vi "setFPGA.vi"(10 "FPGA":refnum<class "FPGA.lvclass">, 11 "ModbusSubnetETxDataFIFO in":refnum<class "ModbusSubnetETxDataFIFO.lvclass">) -> (3 "ModbusSubnetETxDataFIFO out":refnum<class "ModbusSubnetETxDataFIFO.lvclass">)   [LabVIEW 2016, in "ModbusSubnetETxDataFIFO.lvclass"]
uses:
  ModbusSubnetETxDataFIFO.lvclass
  FPGA/FPGA.lvclass
  ModbusSubnetETxDataFIFO.lvclass/ModbusSubnetETxDataFIFO.ctl
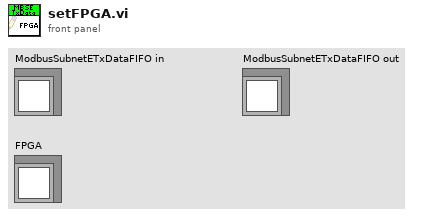
[diagram p1: front panel]
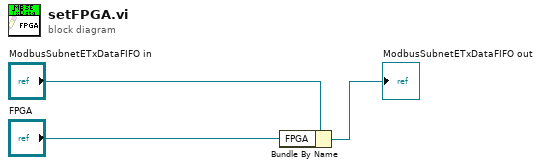
[diagram p0: block diagram]
diagram:
  n1 = Bundle By Name(cluster="ModbusSubnetETxDataFIFO in", "FPGA"="FPGA") -> (→"ModbusSubnetETxDataFIFO out":refnum<class "ModbusSubnetETxDataFIFO.lvclass">)
